vi "Set Led(SubVI).vi"(8 "error in (no error)":errorcluster, 10 "Led Option":T1, 11 "handle in":i64) -> (0 "error out":errorcluster, 3 "handle out":i64)   [LabVIEW 2017]
uses:
  Led Control.ctl
  libkinect_wrapper.dll
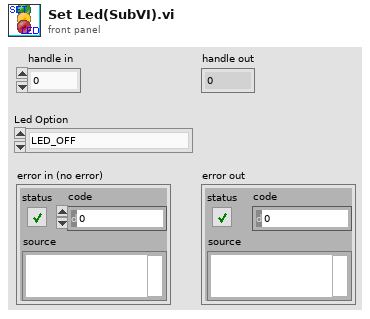
[diagram p1: front panel]
types:
  T1 = typedef "Led Control.ctl" = enum32{"LED_OFF", "LED_GREEN", "LED_RED", "LED_YELLOW", "LED_BLINK_GREEN", "LED_BLINK_GREEN2", "LED_BLINK_RED_YELLOW"}
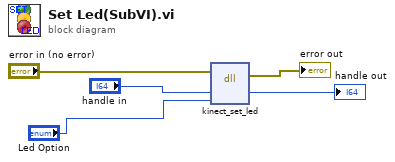
[diagram p0: block diagram]
diagram:
  n1 = dll-call lib="libkinect_wrapper.*" fn="kinect_set_led"(error in="error in (no error)", "handle"="handle in", "option"="Led Option") -> (error out=→"error out":errorcluster, "handle"=→"handle out":i64)  [unwired: 4 in, 1 out]
